vi "Part Change.vi"() -> ()   [LabVIEW 2023]
uses:
  <vilib>/addons/database/Connection.llb/DB Tools Open Connec (String).vi
  <vilib>/regexp/Match Regular Expression.xnode
  <vilib>/addons/database/NI_Database_API.lvlib
panel:
  in  "Reference ID":string
  in  "Type":string(combo)
  in  "Description of Action":string
  in  "Exit":bool
  in  "Enter":bool
  in  "DC_SN":string
  in  "Work Order":string
  in  "Employee Number":string
  # "Part Change"
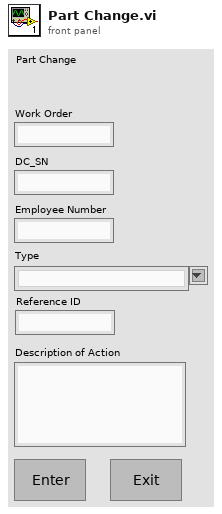
[diagram p1: front panel]
types:
  T1 = typedef "NI_Database_API.lvlib/Conn ObjectReference.ctl" = refnum<k1>
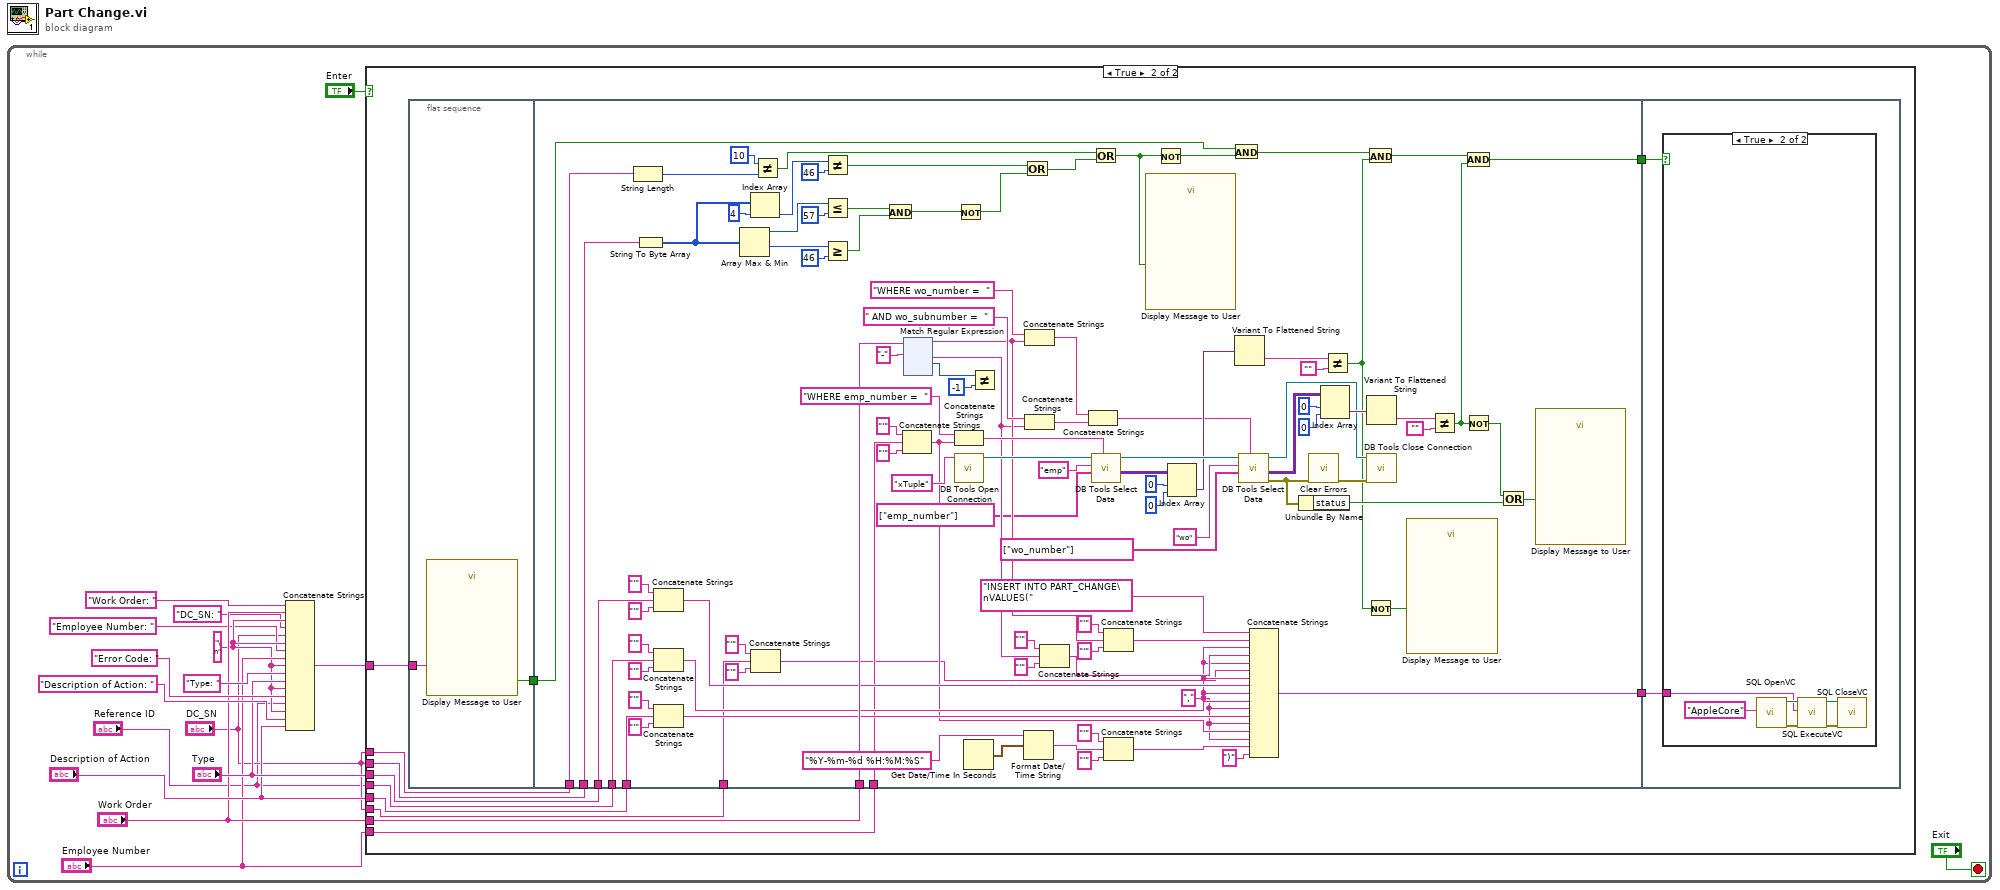
[diagram p0: block diagram]
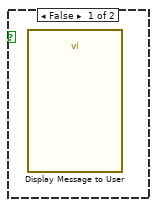
[diagram p3: hidden frame]
diagram:
  n1 = while {
    stop <- "Exit" stop-if-true
    w6 = "\n" ("string")
    n2 = Concatenate Strings("Work Order: " ("string"), "Work Order", w6, "DC_SN: " ("string"), "DC_SN", w6, "Employee Number: " ("string"), "Employee Number", w6, "Type: " ("string"), "Type", w6, "Error Code: " ("string"), "Reference ID", w6, "Description of Action: " ("string"), "Description of Action") -> (w14:string)
    n3 = case shown="True" "Enter" {
      tunnel: w14 -> [_ w28]
      tunnel: "DC_SN" -> [_ w25]
      tunnel: "DC_SN" -> [_ w24]
      tunnel: "Work Order" -> [_ w23]
      tunnel: "Type" -> [_ w21]
      tunnel: "Reference ID" -> [_ w20]
      tunnel: "Description of Action" -> [_ w19]
      tunnel: "Employee Number" -> [_ w18]
      tunnel: "DC_SN" -> [_ w17]
      frame False {
      }
      frame True {
        n4 = flat-sequence {
          tunnel: [w30] -> w27
          tunnel: w28 -> [w29]
          tunnel: w27 -> [w130]
          tunnel: [w48] -> w26
          tunnel: w25 -> [w132]
          tunnel: w24 -> [w131]
          tunnel: w23 -> [w116]
          tunnel: [w100] -> w22
          tunnel: w21 -> [w86]
          tunnel: w20 -> [w82]
          tunnel: w19 -> [w78]
          tunnel: w18 -> [w74]
          tunnel: w17 -> [w67]
          tunnel: w26 -> [w251]
          tunnel: w22 -> [w250]
          frame #0 {
            n5 = call "Display Message to User"("Message"=w29) -> ("Yes"=w30:bool)  [unwired: 9 in, 1 out]
          }
          frame #1 {
            w63 = "," ("string")
            n6 = String Length(string=w131) -> (length=w38:i32)
            n7 = String To Byte Array(string=w132) -> (unsigned byte array=w41:u8[])
            n8 = Concatenate Strings("'" ("string"), w86, "'" ("string")) -> (w85:string)
            n9 = Concatenate Strings("'" ("string"), w82, "'" ("string")) -> (w81:string)
            n10 = Concatenate Strings("'" ("string"), w78, "'" ("string")) -> (w77:string)
            n11 = Array Max & Min(array=w41) -> (max value=w43:u8, min value=w42:u8)  [unwired: 2 out]
            n12 = Index Array(array=w41, index=4) -> (element=w39:u8)
            n13 = Concatenate Strings("'" ("string"), w67, "'" ("string")) -> (w62:string)
            n14 = Not Equal?(x=10, y=w38) -> (x != y?=w31:bool)
            n15 = Not Equal?(x=w39, y=u8 46) -> (x != y?=w40:bool)
            n16 = Less Or Equal?(x=w43, y=u8 57) -> (x <= y?=w44:bool)
            n17 = Greater Or Equal?(x=w42, y=u8 46) -> (x >= y?=w45:bool)
            n18 = And(x=w44, y=w45) -> (x .and. y?=w46:bool)
            n19 = Concatenate Strings("'" ("string"), w74, "'" ("string")) -> (w70:string)
            n20 = xnode "Match Regular Expression"("input string"=w116, "regular expression"="-") -> ("before match"=w93:string, "after match"=w91:string, "offset past match"=w61:i32)  [unwired: 4 in, 2 out]
            n21 = Concatenate Strings("WHERE emp_number =  " ("condition"), w70) -> (w120:string)
            n22 = call-poly <vilib>:"DB Tools Open Connection.vi"("connection information"="xTuple" ("Connection Strings")) -> ("connection reference"=w119:T1)  [unwired: 7 in, 1 out]
            n23 = Not(x=w46) -> (.not. x?=w47:bool)
            n24 = Get Date/Time In Seconds() -> (seconds since 1Jan1904=w98:timestamp)
            n25 = Not Equal?(x=w61, y=-1) -> ()  [unwired: 1 out]
            n26 = Or(x=w40, y=w47) -> (x .or. y?=w32:bool)
            n27 = Format Date/Time String(time format string (%c)="%Y-%m-%d %H:%M:%S", seconds (now)=w98) -> (date/time string=w99:string)  [unwired: 1 in]
            n28 = Concatenate Strings("WHERE wo_number =  " ("condition"), w93) -> (w56:string)
            n29 = Concatenate Strings(" AND wo_subnumber =  " ("condition"), w91) -> (w57:string)
            n30 = Concatenate Strings("'" ("string"), w91, "'" ("string")) -> (w64:string)
            n31 = Concatenate Strings(w56, w57) -> (w58:string)
            n32 = Or(x=w31, y=w32) -> (x .or. y?=w59:bool)
            n33 = call <vilib>:"DB Tools Select Data.vi"("condition"=w120, "columns"=string[] ["emp_number"], "table"="emp", "connection reference"=w119) -> ("data"=w122:variant[][], "connection reference out"=w125:T1)  [unwired: 2 in, 1 out]
            n34 = Concatenate Strings("'" ("string"), w93, "'" ("string")) -> (w65:string)
            n35 = Concatenate Strings("'" ("string"), w99, "'" ("string")) -> (w73:string)
            n36 = call "Display Message to User"("Enable"=w59) -> ()  [unwired: 9 in, 2 out]
            n37 = Not(x=w59) -> (.not. x?=w129:bool)
            n38 = Index Array(array=w122, index (row)=0, index (col)=0 ("disabled index (col)")) -> (element=w121:variant)
            n39 = And(x=w130, y=w129) -> (x .and. y?=w103:bool)
            n40 = Variant To Flattened String(Variant=w121) -> (data string=w123:string)  [unwired: 1 out]
            n41 = call <vilib>:"DB Tools Select Data.vi"("condition"=w58, "columns"=string[] ["wo_number"], "table"="wo", "connection reference"=w125) -> ("error out"=w54:errorcluster, "data"=w128:variant[][], "connection reference out"=w55:T1)  [unwired: 2 in]
            n42 = Concatenate Strings("INSERT INTO PART_CHANGE\nVALUES(" ("string"), w65, w63, w64, w63, w62, w63, w85, w63, w81, w63, w77, w63, w70, w63, w73, ")" ("string")) -> (w100:string)
            n43 = Unbundle By Name(w54) -> ("status"=w51:bool)
            n44 = call <vilib>:"Clear Errors.vi"("error in (no error)"=w54) -> ("error out"=w53:errorcluster)  [unwired: 5 in, 1 out]
            n45 = Index Array(array=w128, index (row)=0, index (col)=0 ("disabled index (col)")) -> (element=w126:variant)
            n46 = Not Equal?(x=w123, y="") -> (x != y?=w49:bool)
            n47 = And(x=w103, y=w49) -> (x .and. y?=w102:bool)
            n48 = Not(x=w49) -> (.not. x?=w124:bool)
            n49 = Variant To Flattened String(Variant=w126) -> (data string=w127:string)  [unwired: 1 out]
            n50 = call <vilib>:"DB Tools Close Connection.vi"("error in (no error)"=w53, "connection reference"=w55) -> ()  [unwired: 5 in, 1 out]
            n51 = call "Display Message to User"("Enable"=w124) -> ()  [unwired: 9 in, 2 out]
            n52 = Not Equal?(x=w127, y="") -> (x != y?=w101:bool)
            n53 = And(x=w102, y=w101) -> (x .and. y?=w48:bool)
            n54 = Not(x=w101) -> (.not. x?=w52:bool)
            n55 = Or(x=w52, y=w51) -> (x .or. y?=w50:bool)
            n56 = call "Display Message to User"("Enable"=w50) -> ()  [unwired: 9 in, 2 out]
          }
          frame #2 {
            n57 = case shown="True" w251 {
              tunnel: w250 -> [_ w252]
              frame False {
                n58 = call "Display Message to User"() -> ()  [unwired: 10 in, 2 out]
              }
              frame True {
                n59 = call "SQL OpenVC.vi"("ConnectionString In"="AppleCore") -> ("Connection Out"=w257:refnum<k7>, "Error out"=w256:errorcluster)  [unwired: 17 in]
                n60 = call "SQL ExecuteVC.vi"("Connection In"=w257, "SQL Query"=w252, "Error in (no error)"=w256) -> ("Connection Out"=w255:refnum<k7>, "Error out"=w254:errorcluster)  [unwired: 15 in]
                n61 = call "SQL CloseVC.vi"("Connection In"=w255, "Error in (no error)"=w254) -> ()  [unwired: 17 in, 1 out]
              }
            }
          }
        }
      }
    }
  }
